vi "Draw.vi"(8 "error in (no error)":errorcluster, 10 "2D Picture in":picture, 11 "Picture in":refnum<class "Image.lvclass">) -> (0 "error out":errorcluster, 2 "2D Picture out":picture, 3 "Picture out":refnum<class "Image.lvclass">)   [LabVIEW 2021, in "Picture2D.lvlib" / "Image.lvclass"]
uses:
  Image.lvclass
  Point/Point.lvclass
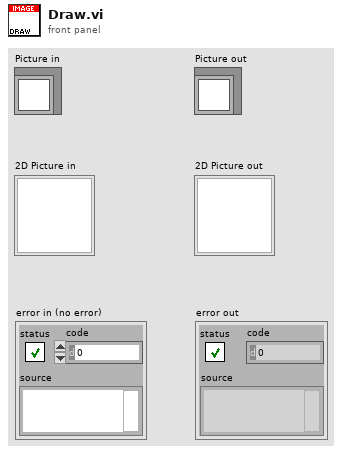
[diagram p1: front panel]
types:
  T1 = typedef "imagedata.ctl" = cluster{"image type":i32, "image depth":i32, "image":u8[], "mask":u8[], "colors":u32[], "Rectangle":cluster{"left":i16, "top":i16, "right":i16, "bottom":i16}}
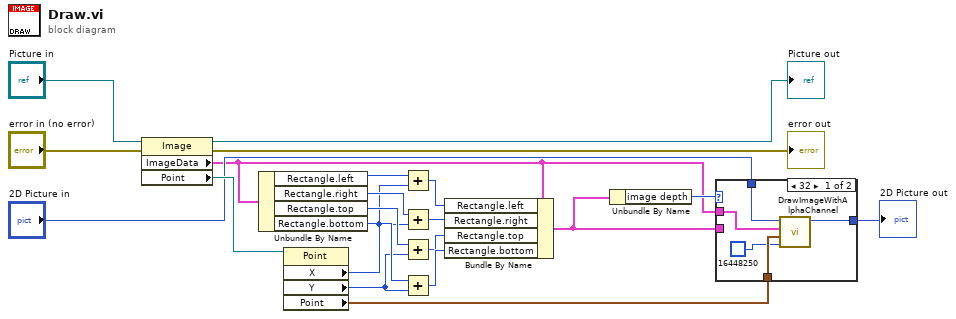
[diagram p0: block diagram]
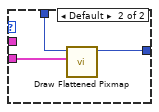
[diagram p2: hidden frame]
diagram:
  n1 = property class="Image"(reference="Picture in", error in="error in (no error)") -> (reference out=→"Picture out":refnum<class "Image.lvclass">, error out=→"error out":errorcluster, "ImageData"=w1:T1, "Point"=w19:refnum<class "Point.lvclass">)
  n2 = Unbundle By Name(w1) -> ("Rectangle.left"=w18:i16, "Rectangle.right"=w15:i16, "Rectangle.top"=w13:i16, "Rectangle.bottom"=w12:i16)
  n3 = property class="Point"(reference=w19) -> ("X"=w8:i16, "Y"=w7:i16, "Point"=w5:cluster{"x":i16, "y":i16})  [unwired: 1 in, 2 out]
  n4 = Add(x=w18, y=w8) -> (x+y=w17:i16)
  n5 = Add(x=w15, y=w8) -> (x+y=w16:i16)
  n6 = Add(x=w13, y=w7) -> (x+y=w11:i16)
  n7 = Add(x=w12, y=w7) -> (x+y=w14:i16)
  n8 = Bundle By Name(cluster=w1, "Rectangle.left"=w17, "Rectangle.right"=w16, "Rectangle.top"=w11, "Rectangle.bottom"=w14) -> (w4:T1)
  n9 = Unbundle By Name(w4) -> ("image depth"=w6:i32)
  n10 = case shown="32" w6 {
    tunnel: w5 -> [w26 _]
    tunnel: w4 -> [_ w28]
    tunnel: "2D Picture in" -> [w25 w27]
    tunnel: [w24 w29] -> w2
    tunnel: w1 -> [w22 _]
    frame 32 {
      n11 = call "DrawImageWithAlphaChannel.vi"("Background Color"=u32 16448250, "Insertion Point (x,y)"=w26, "image data"=w22, "2D Picture in"=w25) -> ("2D Picture out"=w24:picture)  [unwired: 7 in]
    }
    frame Default {
      n12 = call <vilib>:"Draw Flattened Pixmap.vi"("image data"=w28, "picture"=w27) -> ("new picture"=w29:picture)  [unwired: 7 in]
    }
  }
  "2D Picture out" <- w2
